vi "Autonomous Independent.vi"() -> ()   [LabVIEW 2011]
doc: "This VI is called when autonomous begins, and will automatically be terminated when autonomous ends. You can carry out timed or sensor driven robot movement independently without needing to return to the caller."
uses:
  <vilib>/Rock Robotics/WPI/Joystick/WPI_JoystickButtonState.ctl
  Robot Global Data.vi
  <vilib>/addons/control/pid/pid.llb/PID (DBL).vi
  <vilib>/Rock Robotics/WPI/RobotDrive/WPI_RobotDriveArcadeDrive_Standard(NoSaturation).vi
  <vilib>/addons/control/pid/NI_PID_pid.lvlib
panel:
  in  "Initial_Delay_Right":u32(slide)=21 scale=0.0..100.0
  in  "Initial_Delay_Left":u32(slide)=1 scale=0.0..100.0
  in  "Initial_Delay_Center":u32(slide)=1 scale=0.0..100.0
  in  "Ball_Sucker_Right":dbl(slide)=0.6 scale=-1.0..1.0
  in  "Ball_Sucker_Left":dbl(slide)=0.6 scale=-1.0..1.0
  in  "Feed_Speed_Right":dbl(slide)=0.9 scale=-1.0..1.0
  in  "Feed_Speed_Left":dbl(slide)=0.9 scale=-1.0..1.0
  in  "Shooter_Speed_ Right":dbl(slide)=0.65 scale=-1.0..1.0
  in  "Shooter_Speed_Left":dbl(slide)=0.365 scale=-1.0..1.0
  in  "Shooting_Time_Left_Position":u32(slide)=25 scale=0.0..100.0
  in  "Forward_Time1_Left_Position":i32(slide)=45 scale=0.0..100.0
  in  "Backward_Time_Left_Position":i32(slide)=70 scale=0.0..100.0
  in  "Turn_Time_Left_Position":i32(slide)=25 scale=0.0..100.0
  in  "Forward_Time2_Left_Position":i32(slide)=15 scale=0.0..100.0
  in  "Shooting_Time_Right_Position":u32(slide)=35 scale=0.0..100.0
  in  "Forward_Time1_Right_Position":i32(slide)=20 scale=0.0..100.0
  in  "Backward_Time_Right_Position":i32(slide)=81 scale=0.0..100.0
  in  "Turn_Time_Right_Position":i32(slide)=25 scale=0.0..100.0
  in  "Forward_Time2_Right_Position":i32(slide)=15 scale=0.0..100.0
  in  "Forward_Time2_Center_Position":i32(slide)=1 scale=0.0..100.0
  in  "Turn_Time_Center_Position":i32(slide)=1 scale=0.0..100.0
  in  "Backward_Time_Center_Position":i32(slide)=51 scale=0.0..100.0
  in  "Forward_Time1_Center_Position":i32(slide)=51 scale=0.0..100.0
  in  "Shooting_Time_Center_Position":u32(slide)=31 scale=0.0..100.0
  in  "Shooter_Speed_Center":dbl(slide)=0.4 scale=-1.0..1.0
  in  "ARM_FWD_LIMIT":dbl(slide)=0.53 scale=1.0..-1.0
  in  "ARM_REV_LIMIT":dbl(slide)=-0.14110429447852763 scale=1.0..-1.0
  in  "ARM_HOME":dbl(slide)=0.53 scale=1.0..-1.0
  in  "Feeder_Arm_Speed":dbl
  out "JS1_BTNS":T1
  out "JS1_AXES":T2
  in  "Kinect_Arm_Conrol":dbl
  out "Kinect_Drive_Reduce":dbl=0.5
  out "KINECT_BTNS":T1
  out "LEFT_ARM_AXES":T2
  out "RIGHT_ARM_AXES":T2
  in  "Ball_Sucker_Center":dbl(slide)=0.6 scale=-1.0..1.0
  in  "Feed_Speed_Center":dbl(slide)=0.9 scale=-1.0..1.0
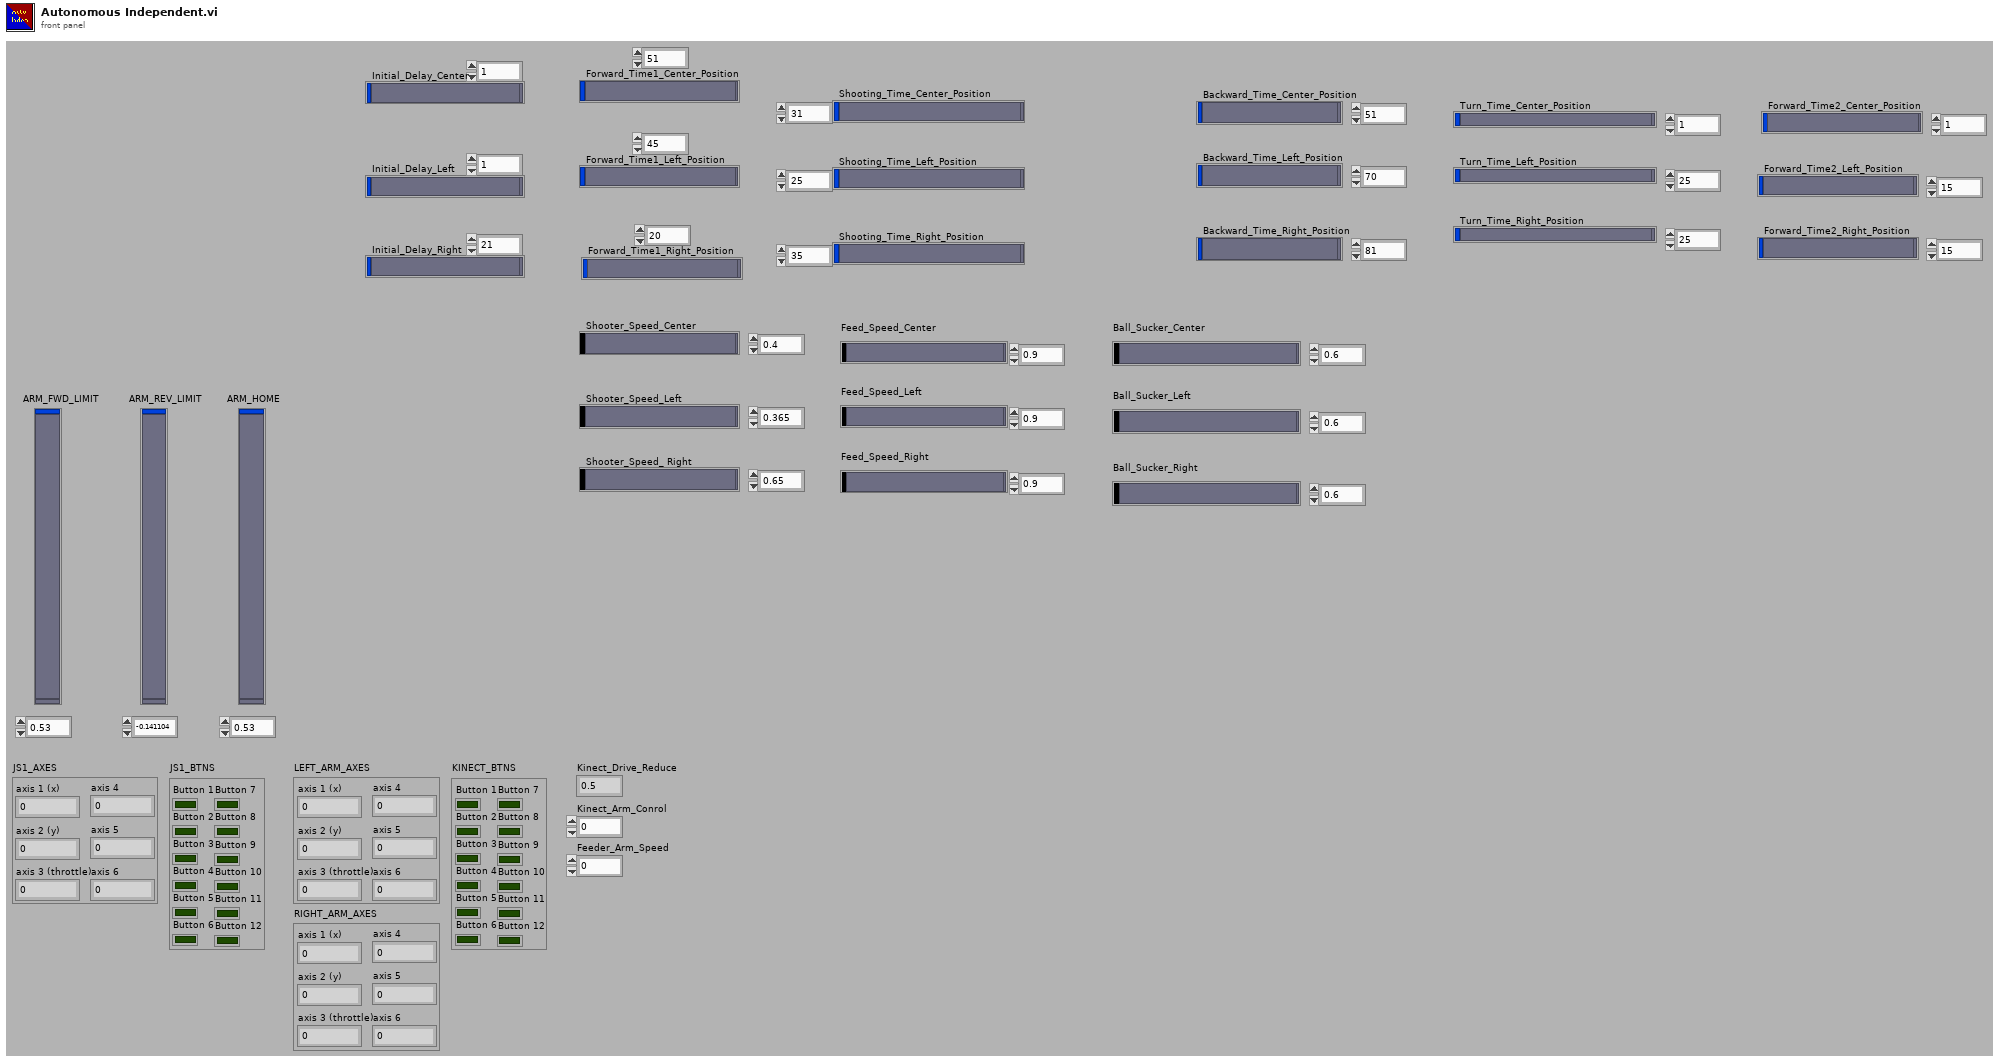
[diagram p1: front panel]
types:
  T1 = typedef "WPI_JoystickButtonState.ctl" = cluster{"Button 1":bool, "Button 2":bool, "Button 3":bool, "Button 4":bool, "Button 5":bool, "Button 6":bool, "Button 7":bool, "Button 8":bool, "Button 9":bool, "Button 10":bool, "Button 11":bool, "Button 12":bool}
  T2 = cluster{"axis 1 (x)":dbl, "axis 2 (y)":dbl, "axis 3 (throttle)":dbl, "axis 4":dbl, "axis 5":dbl, "axis 6":dbl}
  T3 = cluster{"proportional gain (Kc)":dbl, "integral time (Ti, min)":dbl, "derivative time (Td, min)":dbl}
  T4 = typedef "WPI_MotorControlDeviceRef.ctl" = cluster{"DeviceStatus":errorcluster, "Type":enum16{"PWM", "CAN"}, "PWM":cluster{"Digital Module":T5, "PWM Channel":T6, "DeadBand":T7}, "CAN":cluster{"Device Number":u8, "Control Mode":T8, "Semaphore":T9, "Max Vout":dbl}, "Invert":bool, "TransformRef":T10, "InvTransformRef":T10}
  T5 = typedef "FPGA_TypedefDigitalModule.ctl" = enum16{"Digital Module 1", "Digital Module 2"}
  T6 = typedef "FPGA_DIOPWMChannel.ctl" = enum8{"PWM 1", "PWM 2", "PWM 3", "PWM 4", "PWM 5", "PWM 6", "PWM 7", "PWM 8", "PWM 9", "PWM 10", "Invalid"}
  T7 = typedef "WPI_PWMDeadband.ctl" = cluster{"Name":string, "maxPositivePwm":i32, "minPositivePwm":i32, "centerPwm":i32, "maxNegativePwm":i32, "minNegativePwm":i32, "angularRange":u16}
  T8 = typedef "WPI_CANJaguar_ControlMode.ctl" = enum8{"Percent VBus", "Current", "Speed", "Position", "Voltage"}
  T9 = typedef "Semaphore RefNum" = refnum<k1>
  T10 = typedef "WPI_PWMTransform_ConPane.ctl" = refnum<vi>
  T11 = typedef "WPI_RobotDriveDevRef.ctl" = cluster{"DevStatus":errorcluster, "Motors[]":T4[], "Square Inputs":bool, "Max Output":dbl, "Isochronous":bool}
  T12 = typedef "WPI_JoystickDevRef.ctl" = cluster{"Device":T13}
  T13 = typedef "WPI_JoystickDeviceEnum.ctl" = enum16{"USB 1", "USB 2", "USB 3", "USB 4", "Kinect 1", "Kinect 2"}
  T14 = typedef "WPI_AnalogChannelDevRef.ctl" = cluster{"DevStatus":errorcluster, "Analog Module":T15, "Analog Channel":T16}
  T15 = typedef "FPGA_TypedefAnalogModule.ctl" = enum16{"Analog Module 1", "Analog Module 2"}
  T16 = typedef "FPGA_AIChannel.ctl" = enum8{"AI 1", "AI 2", "AI 3", "AI 4", "AI 5", "AI 6", "AI 7", "AI 8", "Invalid"}
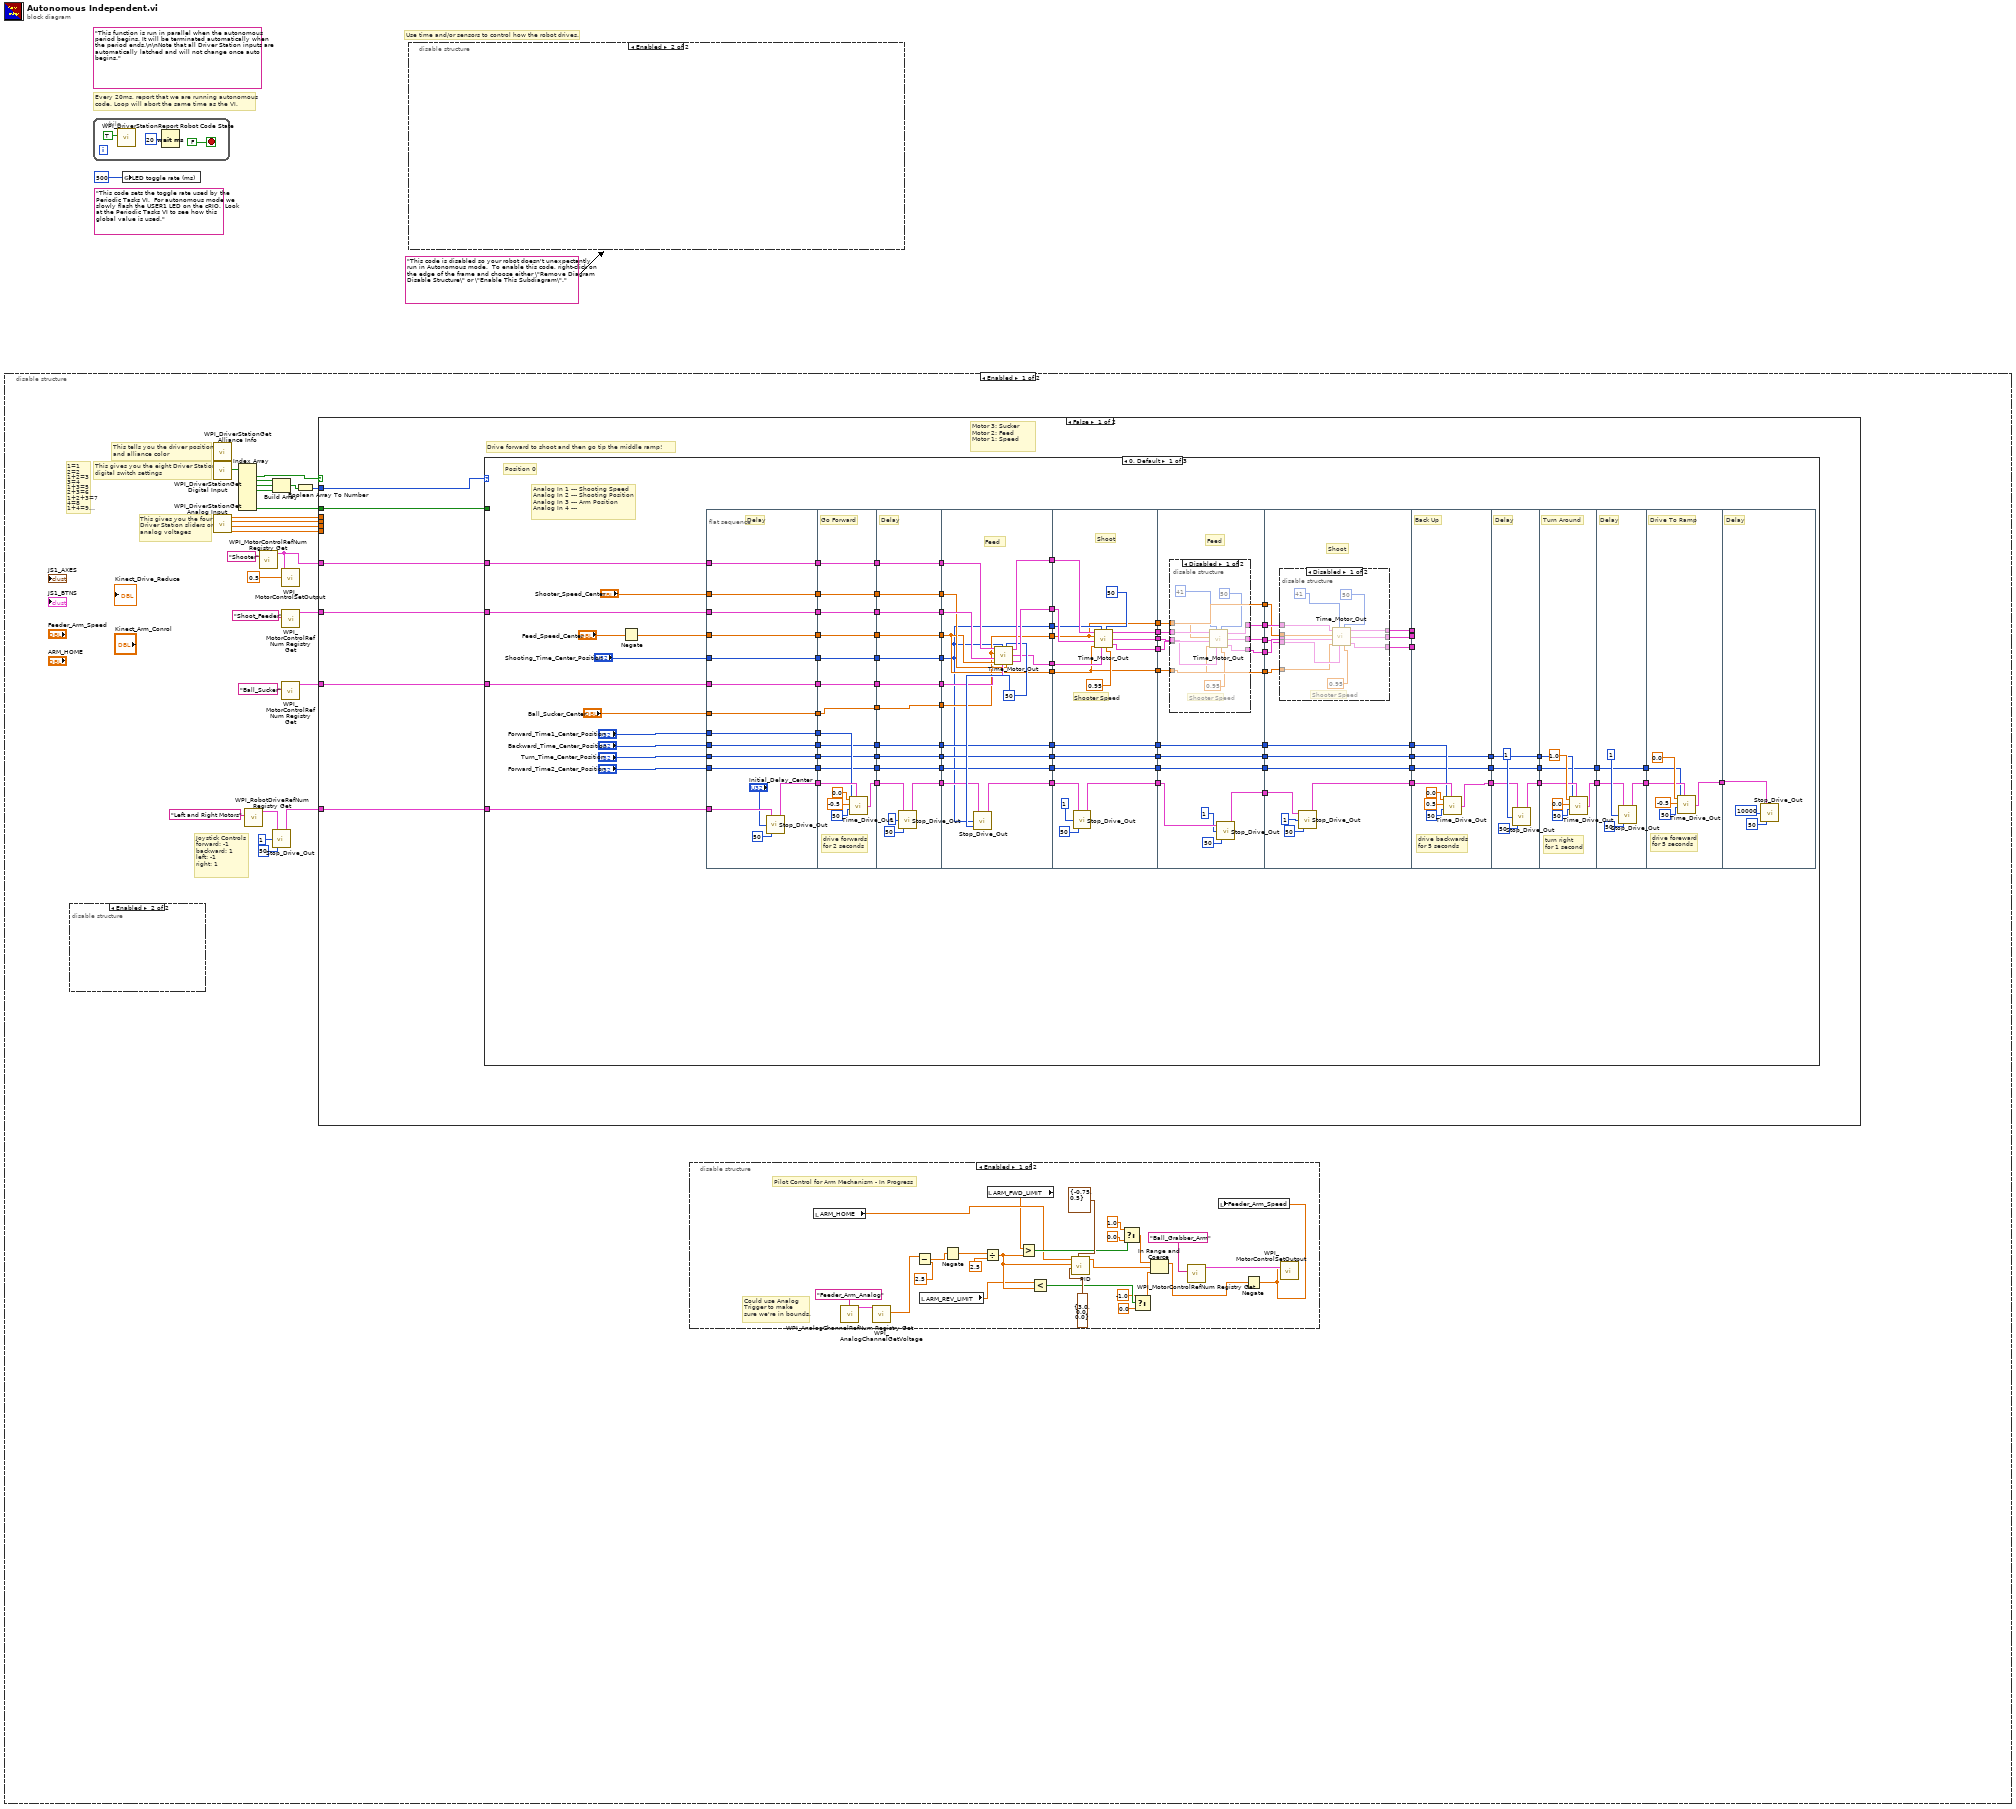
[diagram p0: block diagram]
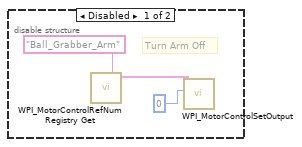
[diagram p3: hidden frame]
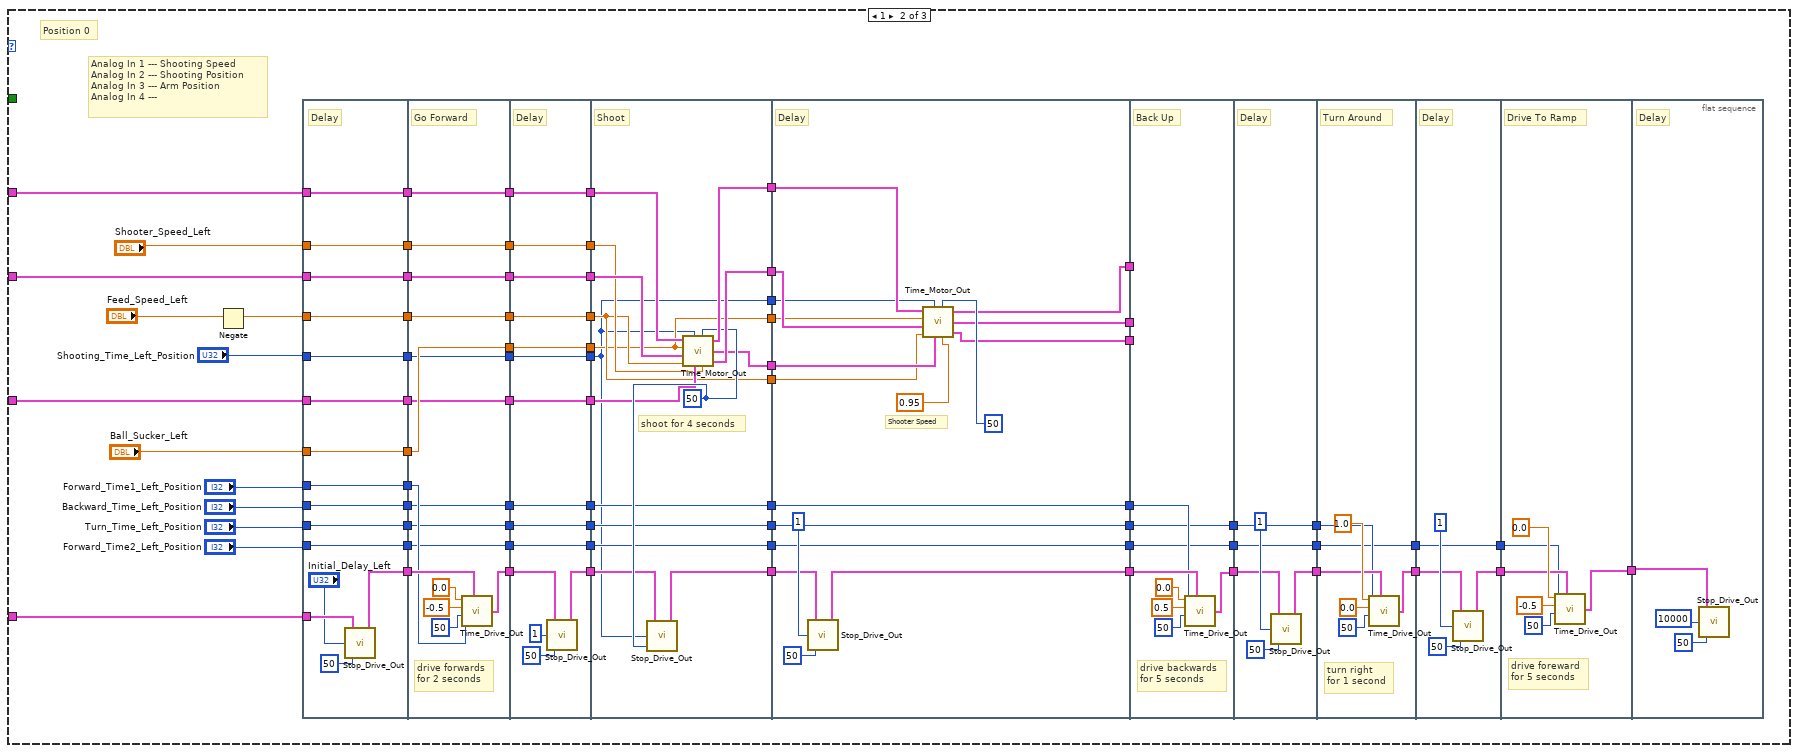
[diagram p6: hidden frame]
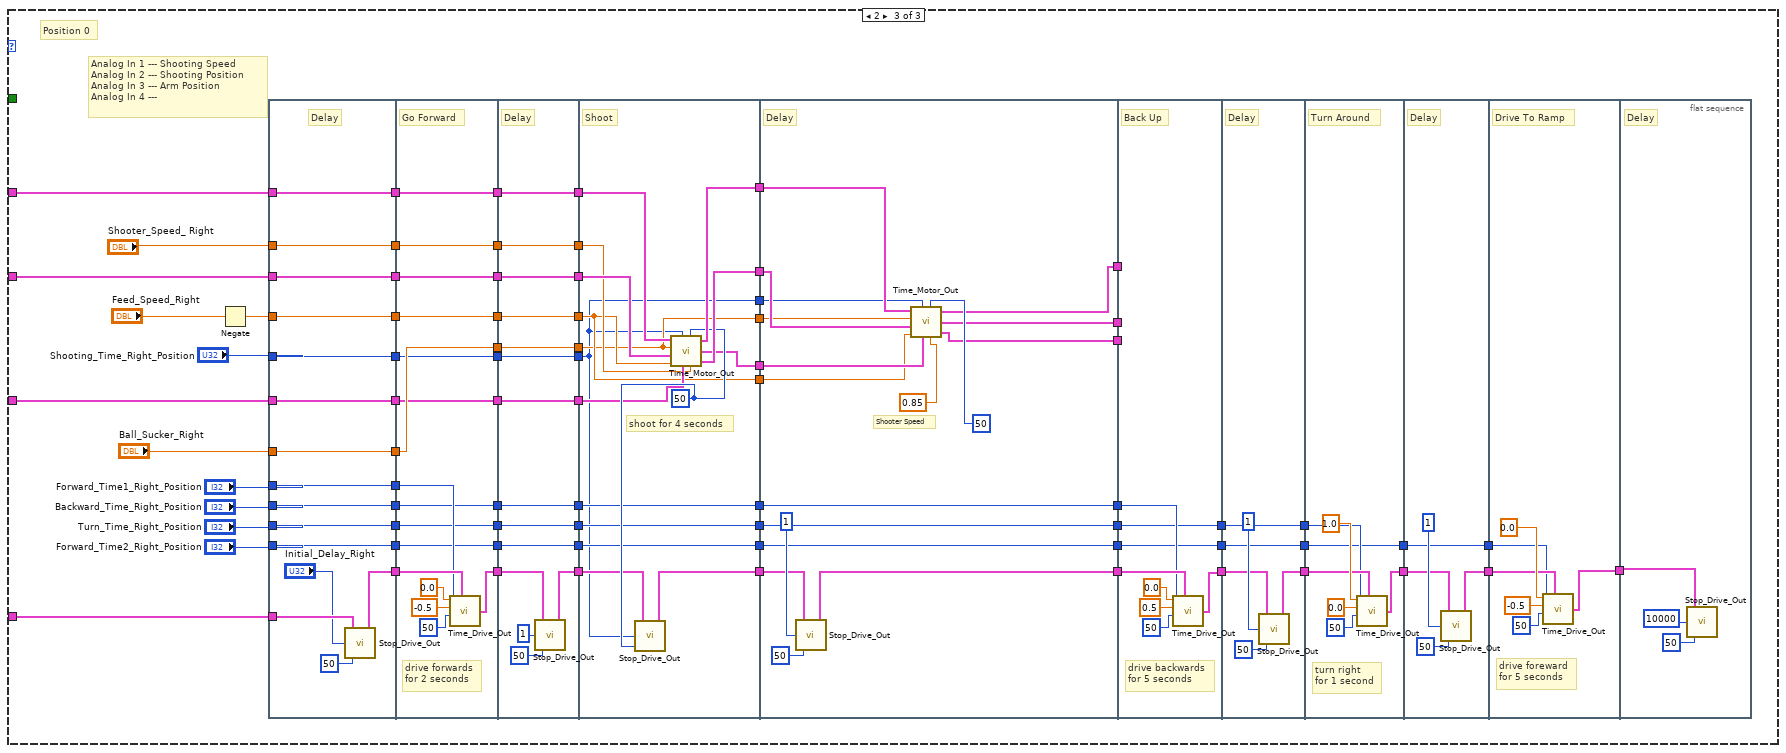
[diagram p7: hidden frame]
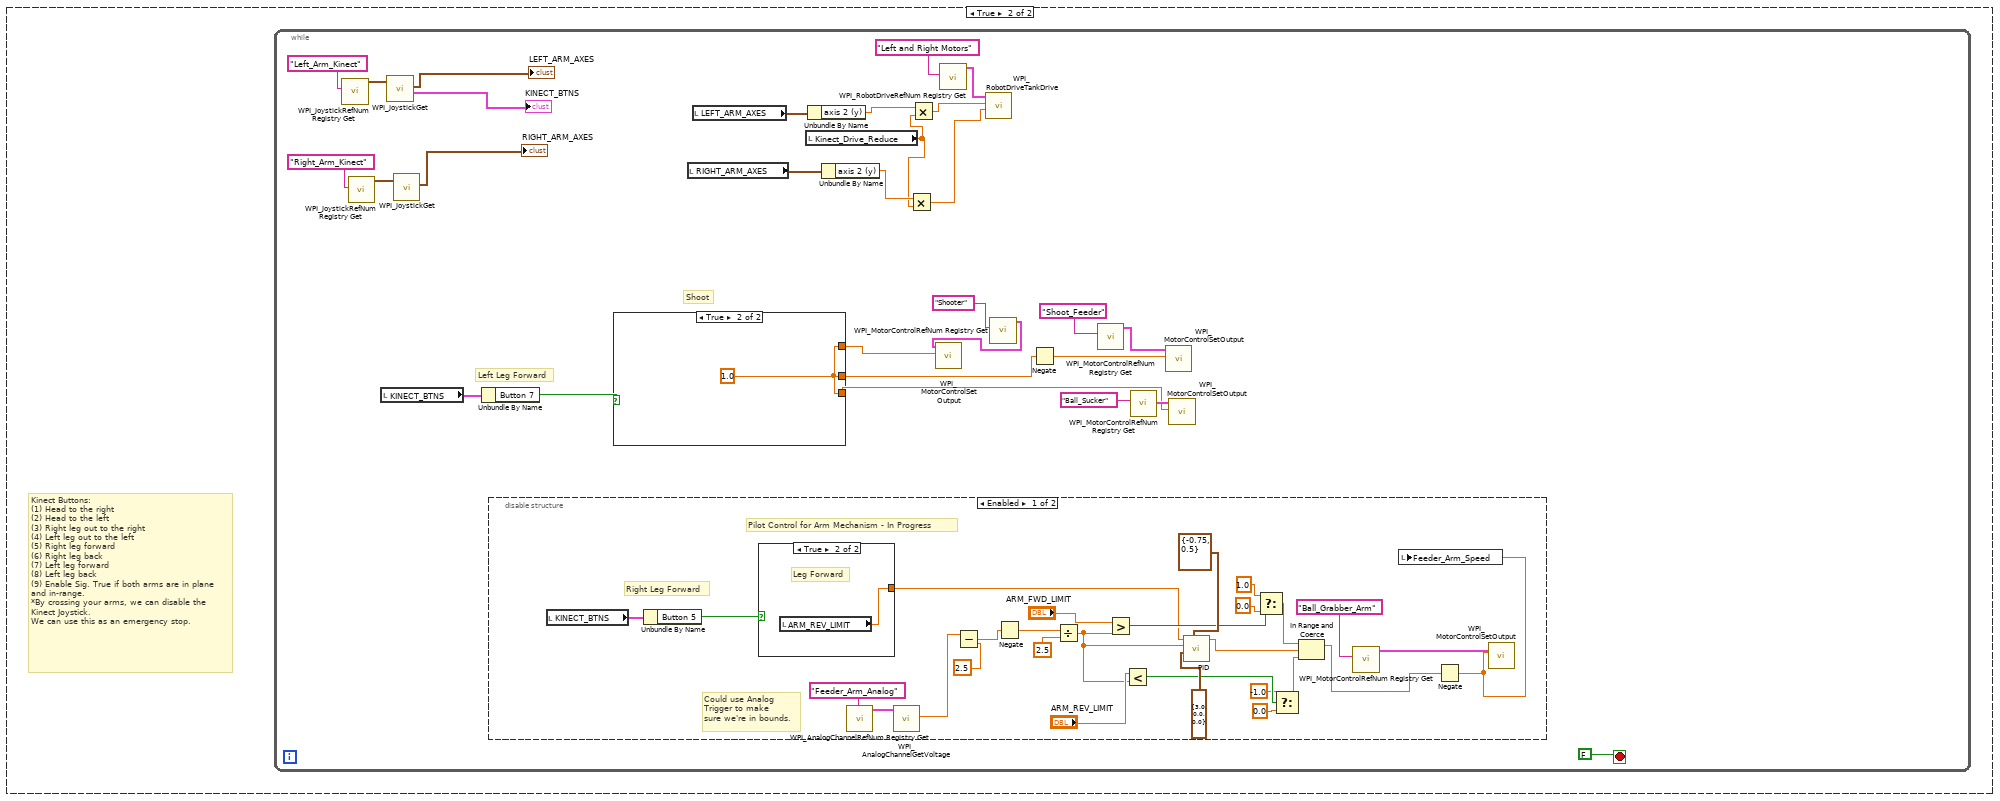
[diagram p8: hidden frame]
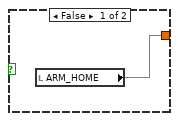
[diagram p9: hidden frame]
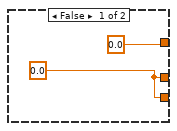
[diagram p11: hidden frame]
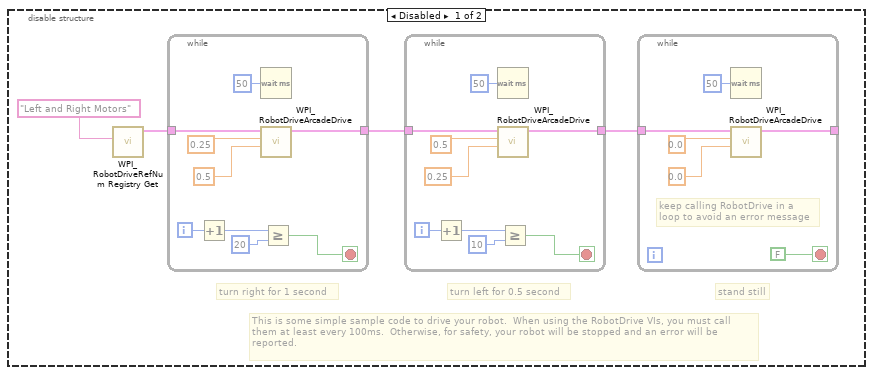
[diagram p13: hidden frame]
diagram:
  (unwired) "This code sets the toggle rate used by the Periodic Tasks VI.  For autonomous mode we slowly flash the USER1 LED on the cRIO.  Look at the Periodic Tasks VI to see how this global value is used."
  (unwired) "This code is disabled so your robot doesn't unexpectantly run in Autonomous mode.  To enable this code, right-click on the edge of the frame and choose either \"Remove Diagram Disable Structure\" or \"Enable This Subdiagram\"."
  (unwired) "This function is run in parallel when the autonomous period begins. It will be terminated automatically when the period ends.\n\nNote that all Driver Station inputs are automatically latched and will not change once auto begins."
  # "Every 20ms, report that we are running autonomous\ncode. Loop will abort the same time as the VI."
  # "Use time and/or sensors to control how the robot drives."
  n1 = disable-structure shown="Enabled" {
    frame Enabled {
      # "Joystick Controls\nforward: -1\nbackward: 1\nleft: -1\nright: 1"
      # "1=1\n2=2\n1+2=3\n3=4\n1+3=5\n2+3=6\n1+2+3=7\n4=8\n1+4=9\n2+4=10\n1+2+4=11\n3+4=12\n1+3+4=13\n2+3+4=14\n1+2+3+4=15"
      # "This tells you the driver position\nand alliance color"
      # "This gives you the eight Driver Station\ndigital switch settings"
      # "This gives you the four\nDriver Station sliders or\nanalog voltages"
      n2 = disable-structure shown="Enabled" {
        frame Disabled {
          # "Turn Arm Off"
          n3 = call <vilib>:"WPI_MotorControlRefNum Registry Get.vi"("refnum name"="Ball_Grabber_Arm") -> ("MotorControlDevRef"=w54:T4)  [unwired: 1 in, 9 out]
          n4 = call <vilib>:"WPI_MotorControlSetOutput.vi"("Output"=0, "MotorControlDevRef"=w54) -> ()  [unwired: 3 in, 7 out]
        }
        frame Enabled {
        }
      }
      n5 = call <vilib>:"WPI_DriverStationGet Alliance Info.vi"() -> ()  [unwired: 12 out]
      n6 = call <vilib>:"WPI_DriverStationGet Digital Input.vi"() -> ("Driver Station Digital Input (1-8)"=w25:bool[])  [unwired: 11 out]
      n7 = call <vilib>:"WPI_DriverStationGet Analog Input.vi"() -> ("Analog 4 (V)"=w22:dbl, "Analog 3 (V)"=w23:dbl, "Analog 2 (V)"=w13:dbl, "Analog 1 (V)"=w14:dbl)  [unwired: 8 out]
      n8 = Index Array(array=w25) -> (element #1=w3:bool, element #2=w2:bool, element #3=w16:bool, element #4=w15:bool, element #8=w21:bool)  [unwired: 8 in, 3 out]
      n9 = call <vilib>:"WPI_RobotDriveRefNum Registry Get.vi"("refnum name"="Left and Right Motors") -> ("RobotDriveDevRef"=w10:T11)  [unwired: 1 in, 9 out]
      n10 = call <vilib>:"WPI_MotorControlRefNum Registry Get.vi"("refnum name"="Shooter") -> ("MotorControlDevRef"=w5:T4)  [unwired: 9 in, 1 out]
      n11 = call "Stop_Drive_Out.vi"("Step_Duration_ms"=50, "Num_Steps"=u32 1 ("milliseconds to wait"), "Drive_In"=w10) -> ("Drive_Out"=w9:T11)
      n12 = Build Array(w2, w16, w15) -> (w24:bool[])
      n13 = call <vilib>:"WPI_MotorControlSetOutput.vi"("Output"=0.5, "MotorControlDevRef"=w5) -> ()  [unwired: 8 in, 2 out]
      n14 = call <vilib>:"WPI_MotorControlRefNum Registry Get.vi"("refnum name"="Ball_Sucker") -> ("MotorControlDevRef"=w6:T4)  [unwired: 9 in, 1 out]
      n15 = call <vilib>:"WPI_MotorControlRefNum Registry Get.vi"("refnum name"="Shoot_Feeder") -> ("MotorControlDevRef"=w18:T4)  [unwired: 9 in, 1 out]
      n16 = Boolean Array To Number(Boolean array=w24) -> (number=w8:u32)
      n17 = case shown="False" w3 {
        tunnel: w14 -> [_ _]
        tunnel: w13 -> [_ _]
        tunnel: w23 -> [_ _]
        tunnel: w22 -> [_ _]
        tunnel: w21 -> [w60 _]
        tunnel: w5 -> [w59 _]
        tunnel: w18 -> [w58 _]
        tunnel: w9 -> [w57 _]
        tunnel: w8 -> [w56 _]
        tunnel: w6 -> [w55 _]
        frame False {
          # "Motor 3: Sucker\nMotor 2: Feed\nMotor 1: Speed"
          # "Drive forward to shoot and then go tip the middle ramp!"
          n18 = case shown="0, Default" w56 {
            tunnel: w60 -> [_ _ _]
            tunnel: w59 -> [w153 w394 w583]
            tunnel: w58 -> [w152 w393 w582]
            tunnel: w57 -> [w151 w392 w581]
            tunnel: w55 -> [w150 w391 w580]
            frame 0, Default {
              # "Analog In 1 --- Shooting Speed\nAnalog In 2 --- Shooting Position\nAnalog In 3 --- Arm Position\nAnalog In 4 ---"
              # "Position 0"
              n19 = Negate(x="Feed_Speed_Center") -> (-x=w88:dbl)
              n20 = flat-sequence {
                tunnel: [w163] -> w149
                tunnel: [w168] -> w148
                tunnel: [w167] -> w147
                tunnel: [w166] -> w146
                tunnel: [w165] -> w145
                tunnel: w153 -> [w166]
                tunnel: w152 -> [w167]
                tunnel: "Shooter_Speed_Center" -> [w165]
                tunnel: w88 -> [w168]
                tunnel: w151 -> [w162]
                tunnel: [w161] -> w144
                tunnel: "Ball_Sucker_Center" -> [w161]
                tunnel: [w160] -> w143
                tunnel: w150 -> [w160]
                tunnel: [w158] -> w117
                tunnel: "Shooting_Time_Center_Position" -> [w158]
                tunnel: "Forward_Time1_Center_Position" -> [w157]
                tunnel: [w157] -> w116
                tunnel: "Backward_Time_Center_Position" -> [w156]
                tunnel: [w156] -> w115
                tunnel: "Turn_Time_Center_Position" -> [w155]
                tunnel: [w155] -> w106
                tunnel: [w154] -> w103
                tunnel: "Forward_Time2_Center_Position" -> [w154]
                tunnel: w149 -> [w181]
                tunnel: [w180] -> w142
                tunnel: [w179] -> w141
                tunnel: w148 -> [w179]
                tunnel: [w178] -> w140
                tunnel: w147 -> [w178]
                tunnel: [w177] -> w139
                tunnel: w146 -> [w177]
                tunnel: [w176] -> w138
                tunnel: w145 -> [w176]
                tunnel: w144 -> [w175]
                tunnel: [w175] -> w137
                tunnel: w143 -> [w174]
                tunnel: [w174] -> w136
                tunnel: [w173] -> w118
                tunnel: w117 -> [w173]
                tunnel: w116 -> [w172]
                tunnel: w115 -> [w171]
                tunnel: [w171] -> w114
                tunnel: [w170] -> w107
                tunnel: w106 -> [w170]
                tunnel: [w169] -> w104
                tunnel: w103 -> [w169]
                tunnel: w142 -> [w192]
                tunnel: [w191] -> w135
                tunnel: [w198] -> w134
                tunnel: w141 -> [w198]
                tunnel: [w197] -> w133
                tunnel: w140 -> [w197]
                tunnel: [w196] -> w132
                tunnel: w139 -> [w196]
                tunnel: [w195] -> w131
                tunnel: w138 -> [w195]
                tunnel: [w190] -> w130
                tunnel: w137 -> [w190]
                tunnel: [w189] -> w129
                tunnel: w136 -> [w189]
                tunnel: [w188] -> w119
                tunnel: w118 -> [w188]
                tunnel: w114 -> [w187]
                tunnel: [w187] -> w113
                tunnel: [w186] -> w108
                tunnel: w107 -> [w186]
                tunnel: [w185] -> w105
                tunnel: w104 -> [w185]
                tunnel: w135 -> [w209]
                tunnel: [w208] -> w128
                tunnel: w134 -> [w201]
                tunnel: w133 -> [w214]
                tunnel: [w213] -> w127
                tunnel: [w212] -> w126
                tunnel: w132 -> [w211]
                tunnel: w131 -> [w205]
                tunnel: [w207] -> w125
                tunnel: w130 -> [w200]
                tunnel: w129 -> [w206]
                tunnel: w119 -> [w199]
                tunnel: w113 -> [w204]
                tunnel: [w204] -> w112
                tunnel: [w203] -> w109
                tunnel: w108 -> [w203]
                tunnel: w105 -> [w202]
                tunnel: [w202] -> w98
                tunnel: [w201] -> w92
                tunnel: [w200] -> w91
                tunnel: [w199] -> w90
                tunnel: w128 -> [w230]
                tunnel: [w229] -> w85
                tunnel: w127 -> [w223]
                tunnel: w126 -> [w224]
                tunnel: w125 -> [w222]
                tunnel: w112 -> [w228]
                tunnel: [w228] -> w84
                tunnel: [w227] -> w83
                tunnel: w109 -> [w227]
                tunnel: [w226] -> w82
                tunnel: w98 -> [w226]
                tunnel: [w221] -> w81
                tunnel: [w220] -> w80
                tunnel: w92 -> [w216]
                tunnel: w91 -> [w215]
                tunnel: w90 -> [w219]
                tunnel: [w217] -> w71
                tunnel: [w216] -> w64
                tunnel: [w215] -> w62
                tunnel: w85 -> [w243]
                tunnel: w84 -> [w247]
                tunnel: [w247] -> w78
                tunnel: w83 -> [w246]
                tunnel: [w246] -> w76
                tunnel: w82 -> [w245]
                tunnel: [w245] -> w74
                tunnel: w81 -> [w235]
                tunnel: w80 -> [w239]
                tunnel: [w241] -> w72
                tunnel: w71 -> [w240]
                tunnel: [w238] -> w70
                tunnel: [w237] -> w69
                tunnel: [w236] -> w68
                tunnel: w64 -> [w234]
                tunnel: [w234] -> w63
                tunnel: w62 -> [w233]
                tunnel: [w233] -> w61
                tunnel: [w268] -> w79
                tunnel: w78 -> [w273]
                tunnel: [w273] -> w77
                tunnel: w76 -> [w272]
                tunnel: [w272] -> w75
                tunnel: w74 -> [w271]
                tunnel: [w271] -> w73
                tunnel: w72 -> [w269]
                tunnel: w70 -> [w266]
                tunnel: w69 -> [w264]
                tunnel: w68 -> [w265]
                tunnel: [w263] -> w67
                tunnel: [w262] -> w66
                tunnel: [w261] -> w65
                tunnel: w63 -> [w260]
                tunnel: w61 -> [w259]
                tunnel: w79 -> [w289]
                tunnel: [w288] -> w124
                tunnel: w77 -> [w287]
                tunnel: [w286] -> w110
                tunnel: w75 -> [w286]
                tunnel: [w285] -> w99
                tunnel: w73 -> [w285]
                tunnel: w67 -> [_]
                tunnel: w66 -> [_]
                tunnel: w65 -> [_]
                tunnel: w124 -> [w296]
                tunnel: [w295] -> w123
                tunnel: [w294] -> w111
                tunnel: w110 -> [w294]
                tunnel: [w293] -> w100
                tunnel: w99 -> [w293]
                tunnel: [w301] -> w122
                tunnel: w123 -> [w302]
                tunnel: w111 -> [w300]
                tunnel: [w299] -> w101
                tunnel: w100 -> [w299]
                tunnel: w122 -> [w308]
                tunnel: [w307] -> w121
                tunnel: [w306] -> w102
                tunnel: w101 -> [w306]
                tunnel: w121 -> [w313]
                tunnel: [w312] -> w120
                tunnel: w102 -> [w311]
                tunnel: w120 -> [w317]
                frame #0 {
                  # "Delay"
                  n21 = call "Stop_Drive_Out.vi"("Step_Duration_ms"=50, "Num_Steps"="Initial_Delay_Center", "Drive_In"=w162) -> ("Drive_Out"=w163:T11)
                }
                frame #1 {
                  # "drive forwards\nfor 2 seconds"
                  # "Go Forward"
                  n22 = call "Time_Drive_Out.vi"("X_Axis"=0.0 ("X axis value"), "Y_Axis"=-0.5 ("X axis value"), "Step_Duration_ms"=u32 50 ("milliseconds to wait"), "Num_Steps"=w172, "Drive_In"=w181) -> ("Drive_Out"=w180:T11)
                }
                frame #2 {
                  # "Delay"
                  n23 = call "Stop_Drive_Out.vi"("Step_Duration_ms"=50, "Num_Steps"=u32 1 ("milliseconds to wait"), "Drive_In"=w192) -> ("Drive_Out"=w191:T11)
                }
                frame #3 {
                  w210 = 50
                  # "Feed"
                  n24 = call "Stop_Drive_Out.vi"("Step_Duration_ms"=w210, "Num_Steps"=w199, "Drive_In"=w209) -> ("Drive_Out"=w208:T11)
                  n25 = call "Time_Motor_Out.vi"("Motor_1_Speed"=w205, "Step_Duration_ms"=w210, "Motor_3"=w206, "Motor_2_Speed"=w201, "Motor_2"=w214, "Num_Steps"=w199, "Motor_3_Speed"=w200, "Motor_1"=w211) -> ("Motor_2_Out"=w213:T4, "Motor_3_Out"=w207:T4, "Motor_1_Out"=w212:T4)
                }
                frame #4 {
                  # "Shooter Speed"
                  # "Shoot"
                  n26 = call "Stop_Drive_Out.vi"("Step_Duration_ms"=50, "Num_Steps"=u32 1 ("milliseconds to wait"), "Drive_In"=w230) -> ("Drive_Out"=w229:T11)
                  n27 = call "Time_Motor_Out.vi"("Motor_1_Speed"=0.95, "Step_Duration_ms"=50, "Motor_3"=w222, "Motor_2_Speed"=w216, "Motor_2"=w223, "Num_Steps"=w219, "Motor_3_Speed"=w215, "Motor_1"=w224) -> ("Motor_2_Out"=w220:T4, "Motor_3_Out"=w221:T4, "Motor_1_Out"=w217:T4)
                }
                frame #5 {
                  # "Feed"
                  n28 = disable-structure shown="Disabled" {
                    disable-tunnel: w240 -> [w256 _]
                    disable-tunnel: w239 -> [w255 _]
                    disable-tunnel: [w254 _] -> w238
                    disable-tunnel: [w253 _] -> w237
                    disable-tunnel: [w252 _] -> w236
                    disable-tunnel: w235 -> [w251 _]
                    disable-tunnel: w234 -> [w249 _]
                    disable-tunnel: w233 -> [w248 _]
                    frame Disabled {
                      # "Shooter Speed"
                      n29 = call "Time_Motor_Out.vi"("Motor_1_Speed"=0.95, "Step_Duration_ms"=50, "Motor_3"=w251, "Motor_2_Speed"=w249, "Motor_2"=w255, "Num_Steps"=41, "Motor_3_Speed"=w248, "Motor_1"=w256) -> ("Motor_2_Out"=w252:T4, "Motor_3_Out"=w253:T4, "Motor_1_Out"=w254:T4)
                    }
                    frame Enabled {
                    }
                  }
                  n30 = call "Stop_Drive_Out.vi"("Step_Duration_ms"=50, "Num_Steps"=u32 1 ("milliseconds to wait"), "Drive_In"=w243) -> ("Drive_Out"=w241:T11)
                }
                frame #6 {
                  # "Shoot"
                  n31 = disable-structure shown="Disabled" {
                    disable-tunnel: w266 -> [w282 _]
                    disable-tunnel: w265 -> [w281 _]
                    disable-tunnel: w264 -> [w280 _]
                    disable-tunnel: [w279 _] -> w263
                    disable-tunnel: [w278 _] -> w262
                    disable-tunnel: [w277 _] -> w261
                    disable-tunnel: w260 -> [w275 _]
                    disable-tunnel: w259 -> [w274 _]
                    frame Disabled {
                      # "Shooter Speed"
                      n32 = call "Time_Motor_Out.vi"("Motor_1_Speed"=0.95, "Step_Duration_ms"=50, "Motor_3"=w280, "Motor_2_Speed"=w275, "Motor_2"=w281, "Num_Steps"=41, "Motor_3_Speed"=w274, "Motor_1"=w282) -> ("Motor_2_Out"=w278:T4, "Motor_3_Out"=w279:T4, "Motor_1_Out"=w277:T4)
                    }
                    frame Enabled {
                    }
                  }
                  n33 = call "Stop_Drive_Out.vi"("Step_Duration_ms"=50, "Num_Steps"=u32 1 ("milliseconds to wait"), "Drive_In"=w269) -> ("Drive_Out"=w268:T11)
                }
                frame #7 {
                  # "Back Up"
                  # "drive backwards\nfor 5 seconds"
                  n34 = call "Time_Drive_Out.vi"("X_Axis"=0.0 ("X axis value"), "Y_Axis"=0.5 ("X axis value"), "Step_Duration_ms"=u32 50 ("milliseconds to wait"), "Num_Steps"=w287, "Drive_In"=w289) -> ("Drive_Out"=w288:T11)
                }
                frame #8 {
                  # "Delay"
                  n35 = call "Stop_Drive_Out.vi"("Step_Duration_ms"=50, "Num_Steps"=u32 1 ("milliseconds to wait"), "Drive_In"=w296) -> ("Drive_Out"=w295:T11)
                }
                frame #9 {
                  # "turn right\nfor 1 second"
                  # "Turn Around"
                  n36 = call "Time_Drive_Out.vi"("X_Axis"=1.0 ("X axis value"), "Y_Axis"=0.0 ("X axis value"), "Step_Duration_ms"=u32 50 ("milliseconds to wait"), "Num_Steps"=w300, "Drive_In"=w302) -> ("Drive_Out"=w301:T11)
                }
                frame #10 {
                  # "Delay"
                  n37 = call "Stop_Drive_Out.vi"("Step_Duration_ms"=50, "Num_Steps"=u32 1 ("milliseconds to wait"), "Drive_In"=w308) -> ("Drive_Out"=w307:T11)
                }
                frame #11 {
                  # "drive foreward\nfor 5 seconds"
                  # "Drive To Ramp"
                  n38 = call "Time_Drive_Out.vi"("X_Axis"=0.0 ("X axis value"), "Y_Axis"=-0.5 ("X axis value"), "Step_Duration_ms"=u32 50 ("milliseconds to wait"), "Num_Steps"=w311, "Drive_In"=w313) -> ("Drive_Out"=w312:T11)
                }
                frame #12 {
                  # "Delay"
                  n39 = call "Stop_Drive_Out.vi"("Step_Duration_ms"=50, "Num_Steps"=u32 10000 ("milliseconds to wait"), "Drive_In"=w317) -> ()  [unwired: 1 out]
                }
              }
            }
            frame 1 {
              # "Analog In 1 --- Shooting Speed\nAnalog In 2 --- Shooting Position\nAnalog In 3 --- Arm Position\nAnalog In 4 ---"
              # "Position 0"
              n40 = Negate(x="Feed_Speed_Left") -> (-x=w320:dbl)
              n41 = flat-sequence {
                tunnel: [w404] -> w390
                tunnel: [w409] -> w389
                tunnel: [w408] -> w388
                tunnel: [w407] -> w387
                tunnel: [w406] -> w386
                tunnel: w394 -> [w407]
                tunnel: w393 -> [w408]
                tunnel: "Shooter_Speed_Left" -> [w406]
                tunnel: w320 -> [w409]
                tunnel: w392 -> [w403]
                tunnel: [w402] -> w385
                tunnel: "Ball_Sucker_Left" -> [w402]
                tunnel: [w401] -> w384
                tunnel: w391 -> [w401]
                tunnel: [w400] -> w357
                tunnel: "Shooting_Time_Left_Position" -> [w400]
                tunnel: "Forward_Time1_Left_Position" -> [w399]
                tunnel: [w399] -> w356
                tunnel: "Backward_Time_Left_Position" -> [w398]
                tunnel: [w398] -> w355
                tunnel: "Turn_Time_Left_Position" -> [w397]
                tunnel: [w397] -> w344
                tunnel: [w396] -> w341
                tunnel: "Forward_Time2_Left_Position" -> [w396]
                tunnel: w390 -> [w422]
                tunnel: [w421] -> w383
                tunnel: [w420] -> w382
                tunnel: w389 -> [w420]
                tunnel: [w419] -> w381
                tunnel: w388 -> [w419]
                tunnel: [w418] -> w380
                tunnel: w387 -> [w418]
                tunnel: [w417] -> w379
                tunnel: w386 -> [w417]
                tunnel: w385 -> [w416]
                tunnel: [w416] -> w378
                tunnel: w384 -> [w415]
                tunnel: [w415] -> w377
                tunnel: [w414] -> w358
                tunnel: w357 -> [w414]
                tunnel: w356 -> [w413]
                tunnel: w355 -> [w412]
                tunnel: [w412] -> w354
                tunnel: [w411] -> w345
                tunnel: w344 -> [w411]
                tunnel: [w410] -> w342
                tunnel: w341 -> [w410]
                tunnel: w383 -> [w433]
                tunnel: [w432] -> w376
                tunnel: [w439] -> w375
                tunnel: w382 -> [w439]
                tunnel: [w438] -> w374
                tunnel: w381 -> [w438]
                tunnel: [w437] -> w373
                tunnel: w380 -> [w437]
                tunnel: [w436] -> w372
                tunnel: w379 -> [w436]
                tunnel: [w431] -> w371
                tunnel: w378 -> [w431]
                tunnel: [w430] -> w370
                tunnel: w377 -> [w430]
                tunnel: [w429] -> w359
                tunnel: w358 -> [w429]
                tunnel: w354 -> [w428]
                tunnel: [w428] -> w353
                tunnel: [w427] -> w346
                tunnel: w345 -> [w427]
                tunnel: [w426] -> w343
                tunnel: w342 -> [w426]
                tunnel: w376 -> [w450]
                tunnel: [w449] -> w369
                tunnel: w375 -> [w442]
                tunnel: w374 -> [w455]
                tunnel: [w454] -> w368
                tunnel: [w453] -> w367
                tunnel: w373 -> [w452]
                tunnel: w372 -> [w446]
                tunnel: [w448] -> w366
                tunnel: w371 -> [w441]
                tunnel: w370 -> [w447]
                tunnel: w359 -> [w440]
                tunnel: w353 -> [w445]
                tunnel: [w445] -> w352
                tunnel: [w444] -> w347
                tunnel: w346 -> [w444]
                tunnel: w343 -> [w443]
                tunnel: [w443] -> w335
                tunnel: [w442] -> w326
                tunnel: [w441] -> w325
                tunnel: [w440] -> w324
                tunnel: w369 -> [w471]
                tunnel: [w470] -> w365
                tunnel: w368 -> [w464]
                tunnel: w367 -> [w465]
                tunnel: w366 -> [w463]
                tunnel: w352 -> [w469]
                tunnel: [w469] -> w351
                tunnel: [w468] -> w348
                tunnel: w347 -> [w468]
                tunnel: [w467] -> w336
                tunnel: w335 -> [w467]
                tunnel: [w462] -> w329
                tunnel: [w461] -> w328
                tunnel: [w460] -> w327
                tunnel: w326 -> [w459]
                tunnel: w325 -> [w458]
                tunnel: w324 -> [w457]
                tunnel: w365 -> [w478]
                tunnel: [w477] -> w364
                tunnel: w351 -> [w476]
                tunnel: [w475] -> w349
                tunnel: w348 -> [w475]
                tunnel: [w474] -> w337
                tunnel: w336 -> [w474]
                tunnel: w329 -> [_]
                tunnel: w328 -> [_]
                tunnel: w327 -> [_]
                tunnel: w364 -> [w485]
                tunnel: [w484] -> w363
                tunnel: [w483] -> w350
                tunnel: w349 -> [w483]
                tunnel: [w482] -> w338
                tunnel: w337 -> [w482]
                tunnel: [w490] -> w362
                tunnel: w363 -> [w491]
                tunnel: w350 -> [w489]
                tunnel: [w488] -> w339
                tunnel: w338 -> [w488]
                tunnel: w362 -> [w497]
                tunnel: [w496] -> w361
                tunnel: [w495] -> w340
                tunnel: w339 -> [w495]
                tunnel: w361 -> [w502]
                tunnel: [w501] -> w360
                tunnel: w340 -> [w500]
                tunnel: w360 -> [w506]
                frame #0 {
                  # "Delay"
                  n42 = call "Stop_Drive_Out.vi"("Step_Duration_ms"=50, "Num_Steps"="Initial_Delay_Left", "Drive_In"=w403) -> ("Drive_Out"=w404:T11)
                }
                frame #1 {
                  # "drive forwards\nfor 2 seconds"
                  # "Go Forward"
                  n43 = call "Time_Drive_Out.vi"("X_Axis"=0.0 ("X axis value"), "Y_Axis"=-0.5 ("X axis value"), "Step_Duration_ms"=u32 50 ("milliseconds to wait"), "Num_Steps"=w413, "Drive_In"=w422) -> ("Drive_Out"=w421:T11)
                }
                frame #2 {
                  # "Delay"
                  n44 = call "Stop_Drive_Out.vi"("Step_Duration_ms"=50, "Num_Steps"=u32 1 ("milliseconds to wait"), "Drive_In"=w433) -> ("Drive_Out"=w432:T11)
                }
                frame #3 {
                  w451 = 50
                  # "Shoot"
                  # "shoot for 4 seconds"
                  n45 = call "Stop_Drive_Out.vi"("Step_Duration_ms"=w451, "Num_Steps"=w440, "Drive_In"=w450) -> ("Drive_Out"=w449:T11)
                  n46 = call "Time_Motor_Out.vi"("Motor_1_Speed"=w446, "Step_Duration_ms"=w451, "Motor_3"=w447, "Motor_2_Speed"=w442, "Motor_2"=w455, "Num_Steps"=w440, "Motor_3_Speed"=w441, "Motor_1"=w452) -> ("Motor_2_Out"=w454:T4, "Motor_3_Out"=w448:T4, "Motor_1_Out"=w453:T4)
                }
                frame #4 {
                  # "Shooter Speed"
                  # "Delay"
                  n47 = call "Stop_Drive_Out.vi"("Step_Duration_ms"=50, "Num_Steps"=u32 1 ("milliseconds to wait"), "Drive_In"=w471) -> ("Drive_Out"=w470:T11)
                  n48 = call "Time_Motor_Out.vi"("Motor_1_Speed"=0.95, "Step_Duration_ms"=50, "Motor_3"=w463, "Motor_2_Speed"=w459, "Motor_2"=w464, "Num_Steps"=w457, "Motor_3_Speed"=w458, "Motor_1"=w465) -> ("Motor_2_Out"=w460:T4, "Motor_3_Out"=w461:T4, "Motor_1_Out"=w462:T4)
                }
                frame #5 {
                  # "Back Up"
                  # "drive backwards\nfor 5 seconds"
                  n49 = call "Time_Drive_Out.vi"("X_Axis"=0.0 ("X axis value"), "Y_Axis"=0.5 ("X axis value"), "Step_Duration_ms"=u32 50 ("milliseconds to wait"), "Num_Steps"=w476, "Drive_In"=w478) -> ("Drive_Out"=w477:T11)
                }
                frame #6 {
                  # "Delay"
                  n50 = call "Stop_Drive_Out.vi"("Step_Duration_ms"=50, "Num_Steps"=u32 1 ("milliseconds to wait"), "Drive_In"=w485) -> ("Drive_Out"=w484:T11)
                }
                frame #7 {
                  # "turn right\nfor 1 second"
                  # "Turn Around"
                  n51 = call "Time_Drive_Out.vi"("X_Axis"=1.0 ("X axis value"), "Y_Axis"=0.0 ("X axis value"), "Step_Duration_ms"=u32 50 ("milliseconds to wait"), "Num_Steps"=w489, "Drive_In"=w491) -> ("Drive_Out"=w490:T11)
                }
                frame #8 {
                  # "Delay"
                  n52 = call "Stop_Drive_Out.vi"("Step_Duration_ms"=50, "Num_Steps"=u32 1 ("milliseconds to wait"), "Drive_In"=w497) -> ("Drive_Out"=w496:T11)
                }
                frame #9 {
                  # "drive foreward\nfor 5 seconds"
                  # "Drive To Ramp"
                  n53 = call "Time_Drive_Out.vi"("X_Axis"=0.0 ("X axis value"), "Y_Axis"=-0.5 ("X axis value"), "Step_Duration_ms"=u32 50 ("milliseconds to wait"), "Num_Steps"=w500, "Drive_In"=w502) -> ("Drive_Out"=w501:T11)
                }
                frame #10 {
                  # "Delay"
                  n54 = call "Stop_Drive_Out.vi"("Step_Duration_ms"=50, "Num_Steps"=u32 10000 ("milliseconds to wait"), "Drive_In"=w506) -> ()  [unwired: 1 out]
                }
              }
            }
            frame 2 {
              # "Analog In 1 --- Shooting Speed\nAnalog In 2 --- Shooting Position\nAnalog In 3 --- Arm Position\nAnalog In 4 ---"
              # "Position 0"
              n55 = Negate(x="Feed_Speed_Right") -> (-x=w510:dbl)
              n56 = flat-sequence {
                tunnel: [w593] -> w579
                tunnel: [w598] -> w578
                tunnel: [w597] -> w577
                tunnel: [w596] -> w576
                tunnel: [w595] -> w575
                tunnel: w583 -> [w596]
                tunnel: w582 -> [w597]
                tunnel: "Shooter_Speed_ Right" -> [w595]
                tunnel: w510 -> [w598]
                tunnel: w581 -> [w592]
                tunnel: [w591] -> w574
                tunnel: "Ball_Sucker_Right" -> [w591]
                tunnel: [w590] -> w573
                tunnel: w580 -> [w590]
                tunnel: [w589] -> w546
                tunnel: "Shooting_Time_Right_Position" -> [w589]
                tunnel: "Forward_Time1_Right_Position" -> [w588]
                tunnel: [w588] -> w545
                tunnel: "Backward_Time_Right_Position" -> [w587]
                tunnel: [w587] -> w544
                tunnel: "Turn_Time_Right_Position" -> [w586]
                tunnel: [w586] -> w533
                tunnel: [w585] -> w530
                tunnel: "Forward_Time2_Right_Position" -> [w585]
                tunnel: w579 -> [w611]
                tunnel: [w610] -> w572
                tunnel: [w609] -> w571
                tunnel: w578 -> [w609]
                tunnel: [w608] -> w570
                tunnel: w577 -> [w608]
                tunnel: [w607] -> w569
                tunnel: w576 -> [w607]
                tunnel: [w606] -> w568
                tunnel: w575 -> [w606]
                tunnel: w574 -> [w605]
                tunnel: [w605] -> w567
                tunnel: w573 -> [w604]
                tunnel: [w604] -> w566
                tunnel: [w603] -> w547
                tunnel: w546 -> [w603]
                tunnel: w545 -> [w602]
                tunnel: w544 -> [w601]
                tunnel: [w601] -> w543
                tunnel: [w600] -> w534
                tunnel: w533 -> [w600]
                tunnel: [w599] -> w531
                tunnel: w530 -> [w599]
                tunnel: w572 -> [w622]
                tunnel: [w621] -> w565
                tunnel: [w628] -> w564
                tunnel: w571 -> [w628]
                tunnel: [w627] -> w563
                tunnel: w570 -> [w627]
                tunnel: [w626] -> w562
                tunnel: w569 -> [w626]
                tunnel: [w625] -> w561
                tunnel: w568 -> [w625]
                tunnel: [w620] -> w560
                tunnel: w567 -> [w620]
                tunnel: [w619] -> w559
                tunnel: w566 -> [w619]
                tunnel: [w618] -> w548
                tunnel: w547 -> [w618]
                tunnel: w543 -> [w617]
                tunnel: [w617] -> w542
                tunnel: [w616] -> w535
                tunnel: w534 -> [w616]
                tunnel: [w615] -> w532
                tunnel: w531 -> [w615]
                tunnel: w565 -> [w639]
                tunnel: [w638] -> w558
                tunnel: w564 -> [w631]
                tunnel: w563 -> [w644]
                tunnel: [w643] -> w557
                tunnel: [w642] -> w556
                tunnel: w562 -> [w641]
                tunnel: w561 -> [w635]
                tunnel: [w637] -> w555
                tunnel: w560 -> [w630]
                tunnel: w559 -> [w636]
                tunnel: w548 -> [w629]
                tunnel: w542 -> [w634]
                tunnel: [w634] -> w541
                tunnel: [w633] -> w536
                tunnel: w535 -> [w633]
                tunnel: w532 -> [w632]
                tunnel: [w632] -> w524
                tunnel: [w631] -> w515
                tunnel: [w630] -> w514
                tunnel: [w629] -> w513
                tunnel: w558 -> [w660]
                tunnel: [w659] -> w554
                tunnel: w557 -> [w653]
                tunnel: w556 -> [w654]
                tunnel: w555 -> [w652]
                tunnel: w541 -> [w658]
                tunnel: [w658] -> w540
                tunnel: [w657] -> w537
                tunnel: w536 -> [w657]
                tunnel: [w656] -> w525
                tunnel: w524 -> [w656]
                tunnel: [w651] -> w518
                tunnel: [w650] -> w517
                tunnel: [w649] -> w516
                tunnel: w515 -> [w648]
                tunnel: w514 -> [w647]
                tunnel: w513 -> [w646]
                tunnel: w554 -> [w667]
                tunnel: [w666] -> w553
                tunnel: w540 -> [w665]
                tunnel: [w664] -> w538
                tunnel: w537 -> [w664]
                tunnel: [w663] -> w526
                tunnel: w525 -> [w663]
                tunnel: w518 -> [_]
                tunnel: w517 -> [_]
                tunnel: w516 -> [_]
                tunnel: w553 -> [w674]
                tunnel: [w673] -> w552
                tunnel: [w672] -> w539
                tunnel: w538 -> [w672]
                tunnel: [w671] -> w527
                tunnel: w526 -> [w671]
                tunnel: [w679] -> w551
                tunnel: w552 -> [w680]
                tunnel: w539 -> [w678]
                tunnel: [w677] -> w528
                tunnel: w527 -> [w677]
                tunnel: w551 -> [w686]
                tunnel: [w685] -> w550
                tunnel: [w684] -> w529
                tunnel: w528 -> [w684]
                tunnel: w550 -> [w691]
                tunnel: [w690] -> w549
                tunnel: w529 -> [w689]
                tunnel: w549 -> [w695]
                frame #0 {
                  # "Delay"
                  n57 = call "Stop_Drive_Out.vi"("Step_Duration_ms"=50, "Num_Steps"="Initial_Delay_Right", "Drive_In"=w592) -> ("Drive_Out"=w593:T11)
                }
                frame #1 {
                  # "drive forwards\nfor 2 seconds"
                  # "Go Forward"
                  n58 = call "Time_Drive_Out.vi"("X_Axis"=0.0 ("X axis value"), "Y_Axis"=-0.5 ("X axis value"), "Step_Duration_ms"=u32 50 ("milliseconds to wait"), "Num_Steps"=w602, "Drive_In"=w611) -> ("Drive_Out"=w610:T11)
                }
                frame #2 {
                  # "Delay"
                  n59 = call "Stop_Drive_Out.vi"("Step_Duration_ms"=50, "Num_Steps"=u32 1 ("milliseconds to wait"), "Drive_In"=w622) -> ("Drive_Out"=w621:T11)
                }
                frame #3 {
                  w640 = 50
                  # "Shoot"
                  # "shoot for 4 seconds"
                  n60 = call "Stop_Drive_Out.vi"("Step_Duration_ms"=w640, "Num_Steps"=w629, "Drive_In"=w639) -> ("Drive_Out"=w638:T11)
                  n61 = call "Time_Motor_Out.vi"("Motor_1_Speed"=w635, "Step_Duration_ms"=w640, "Motor_3"=w636, "Motor_2_Speed"=w631, "Motor_2"=w644, "Num_Steps"=w629, "Motor_3_Speed"=w630, "Motor_1"=w641) -> ("Motor_2_Out"=w643:T4, "Motor_3_Out"=w637:T4, "Motor_1_Out"=w642:T4)
                }
                frame #4 {
                  # "Shooter Speed"
                  # "Delay"
                  n62 = call "Stop_Drive_Out.vi"("Step_Duration_ms"=50, "Num_Steps"=u32 1 ("milliseconds to wait"), "Drive_In"=w660) -> ("Drive_Out"=w659:T11)
                  n63 = call "Time_Motor_Out.vi"("Motor_1_Speed"=0.85, "Step_Duration_ms"=50, "Motor_3"=w652, "Motor_2_Speed"=w648, "Motor_2"=w653, "Num_Steps"=w646, "Motor_3_Speed"=w647, "Motor_1"=w654) -> ("Motor_2_Out"=w649:T4, "Motor_3_Out"=w650:T4, "Motor_1_Out"=w651:T4)
                }
                frame #5 {
                  # "Back Up"
                  # "drive backwards\nfor 5 seconds"
                  n64 = call "Time_Drive_Out.vi"("X_Axis"=0.0 ("X axis value"), "Y_Axis"=0.5 ("X axis value"), "Step_Duration_ms"=u32 50 ("milliseconds to wait"), "Num_Steps"=w665, "Drive_In"=w667) -> ("Drive_Out"=w666:T11)
                }
                frame #6 {
                  # "Delay"
                  n65 = call "Stop_Drive_Out.vi"("Step_Duration_ms"=50, "Num_Steps"=u32 1 ("milliseconds to wait"), "Drive_In"=w674) -> ("Drive_Out"=w673:T11)
                }
                frame #7 {
                  # "turn right\nfor 1 second"
                  # "Turn Around"
                  n66 = call "Time_Drive_Out.vi"("X_Axis"=1.0 ("X axis value"), "Y_Axis"=0.0 ("X axis value"), "Step_Duration_ms"=u32 50 ("milliseconds to wait"), "Num_Steps"=w678, "Drive_In"=w680) -> ("Drive_Out"=w679:T11)
                }
                frame #8 {
                  # "Delay"
                  n67 = call "Stop_Drive_Out.vi"("Step_Duration_ms"=50, "Num_Steps"=u32 1 ("milliseconds to wait"), "Drive_In"=w686) -> ("Drive_Out"=w685:T11)
                }
                frame #9 {
                  # "drive foreward\nfor 5 seconds"
                  # "Drive To Ramp"
                  n68 = call "Time_Drive_Out.vi"("X_Axis"=0.0 ("X axis value"), "Y_Axis"=-0.5 ("X axis value"), "Step_Duration_ms"=u32 50 ("milliseconds to wait"), "Num_Steps"=w689, "Drive_In"=w691) -> ("Drive_Out"=w690:T11)
                }
                frame #10 {
                  # "Delay"
                  n69 = call "Stop_Drive_Out.vi"("Step_Duration_ms"=50, "Num_Steps"=u32 10000 ("milliseconds to wait"), "Drive_In"=w695) -> ()  [unwired: 1 out]
                }
              }
            }
          }
        }
        frame True {
          # "Kinect Buttons:\n(1) Head to the right\n(2) Head to the left\n(3) Right leg out to the right\n(4) Left leg out to the left\n(5) Right leg forward\n(6) Right leg back\n(7) Left leg forward\n(8) Left leg back\n(9) Enable Sig. True if both arms are in plane and in-range.\n*By crossing your arms, we can disable the Kinect Joystick. \nWe can use this as an emergency stop."
          n70 = while {
            stop <- FALSE stop-if-true
            # "Left Leg Forward"
            # "Shoot"
            n71 = call <vilib>:"WPI_JoystickRefNum Registry Get.vi"("refnum name"="Left_Arm_Kinect") -> ("JoystickDevRef"=w723:T12)  [unwired: 1 in, 9 out]
            n72 = call <vilib>:"WPI_JoystickRefNum Registry Get.vi"("refnum name"="Right_Arm_Kinect") -> ("JoystickDevRef"=w721:T12)  [unwired: 1 in, 9 out]
            n73 = local read "KINECT_BTNS"() -> (w711:T1)
            n74 = call <vilib>:"WPI_JoystickGet.vi"("JoystickDevRef"=w723) -> ("Buttons"=→"KINECT_BTNS":T1, "Axes"=→"LEFT_ARM_AXES":T2)  [unwired: 1 in, 4 out]
            n75 = call <vilib>:"WPI_JoystickGet.vi"("JoystickDevRef"=w721) -> ("Axes"=→"RIGHT_ARM_AXES":T2)  [unwired: 1 in, 5 out]
            n76 = Unbundle By Name(w711) -> ("Button 7"=w710:bool)
            n77 = disable-structure shown="Enabled" {
              frame Enabled {
                # "Right Leg Forward"
                # "Could use Analog\nTrigger to make \nsure we're in bounds."
                # "Pilot Control for Arm Mechanism - In Progress"
                n78 = local read "KINECT_BTNS"() -> (w729:T1)
                n79 = Unbundle By Name(w729) -> ("Button 5"=w727:bool)
                n80 = case shown="True" w727 {
                  tunnel: [w755 w756] -> w728
                  frame False {
                    n81 = local read "ARM_HOME"() -> (w755:dbl)
                  }
                  frame True {
                    # "Leg Forward"
                    n82 = local read "ARM_REV_LIMIT"() -> (w756:dbl)
                  }
                }
                n83 = call <vilib>:"WPI_AnalogChannelRefNum Registry Get.vi"("refnum name"="Feeder_Arm_Analog") -> ("AIDeviceRef"=w753:T14)  [unwired: 1 in, 9 out]
                n84 = call <vilib>:"WPI_AnalogChannelGetVoltage.vi"("AIDeviceRef"=w753) -> ("Voltage"=w750:dbl)  [unwired: 1 in, 9 out]
                n85 = Subtract(x=w750, y=2.5) -> (x-y=w733:dbl)
                n86 = Negate(x=w733) -> (-x=w734:dbl)
                n87 = Divide(x=w734, y=2.5) -> (x/y=w731:dbl)
                n88 = Greater?(x="ARM_FWD_LIMIT", y=w731) -> (0:w745:bool)
                n89 = Less?(x="ARM_REV_LIMIT", y=w731) -> (x < y?=w747:bool)
                n90 = call-poly <vilib>:"PID.vi"("output range"=cluster{"output low":dbl, "output high":dbl} {"output low"=-0.75, "output high"=0.5}, "PID gains"=T3 {"proportional gain (Kc)"=3.0, "integral time (Ti, min)"=0.0, "derivative time (Td, min)"=0.0}, "process variable"=w731, "setpoint"=w728) -> ("output"=w738:dbl)  [unwired: 2 in, 5 out]
                n91 = Select(t=1.0, s=w745, f=0.0) -> (s? t:f=w743:dbl)
                n92 = Select(t=-1.0, s=w747, f=0.0) -> (s? t:f=w744:dbl)
                n93 = In Range and Coerce(upper limit=w743, x=w738, lower limit=w744) -> (coerced(x)=w730:dbl)  [unwired: 1 out]
                n94 = call <vilib>:"WPI_MotorControlRefNum Registry Get.vi"("refnum name"="Ball_Grabber_Arm") -> ("MotorControlDevRef"=w754:T4)  [unwired: 1 in, 9 out]
                n95 = Negate(x=w730) -> (-x=w735:dbl)
                n96 = local write "Feeder_Arm_Speed"(w735) -> ()
                n97 = call <vilib>:"WPI_MotorControlSetOutput.vi"("Output"=w735, "MotorControlDevRef"=w754) -> ()  [unwired: 3 in, 7 out]
              }
              frame Disabled {
              }
            }
            n98 = case shown="True" w710 {
              tunnel: [0.0 w759] -> w702
              tunnel: [w758 w759] -> w701
              tunnel: [w758 w759] -> w700
              frame False {
                w758 = 0.0
              }
              frame True {
                w759 = 1.0
              }
            }
            n99 = local read "RIGHT_ARM_AXES"() -> (w714:T2)
            n100 = local read "LEFT_ARM_AXES"() -> (w717:T2)
            n101 = local read "Kinect_Drive_Reduce"() -> (w712:dbl)
            n102 = Unbundle By Name(w717) -> ("axis 2 (y)"=w716:dbl)
            n103 = Unbundle By Name(w714) -> ("axis 2 (y)"=w713:dbl)
            n104 = Multiply(x=w713, y=w712) -> (x*y=w698:dbl)
            n105 = Multiply(x=w716, y=w712) -> (x*y=w715:dbl)
            n106 = call <vilib>:"WPI_RobotDriveRefNum Registry Get.vi"("refnum name"="Left and Right Motors") -> ("RobotDriveDevRef"=w718:T11)  [unwired: 1 in, 9 out]
            n107 = call <vilib>:"WPI_RobotDriveTankDrive.vi"("Right axis value"=w698, "Left axis value"=w715, "RobotDriveDevRef"=w718) -> ()  [unwired: 7 in, 2 out]
            n108 = call <vilib>:"WPI_MotorControlRefNum Registry Get.vi"("refnum name"="Shooter") -> ("MotorControlDevRef"=w708:T4)  [unwired: 9 in, 1 out]
            n109 = call <vilib>:"WPI_MotorControlSetOutput.vi"("Output"=w702, "MotorControlDevRef"=w708) -> ()  [unwired: 8 in, 2 out]
            n110 = Negate(x=w701) -> (-x=w705:dbl)
            n111 = call <vilib>:"WPI_MotorControlRefNum Registry Get.vi"("refnum name"="Shoot_Feeder") -> ("MotorControlDevRef"=w706:T4)  [unwired: 9 in, 1 out]
            n112 = call <vilib>:"WPI_MotorControlRefNum Registry Get.vi"("refnum name"="Ball_Sucker") -> ("MotorControlDevRef"=w703:T4)  [unwired: 9 in, 1 out]
            n113 = call <vilib>:"WPI_MotorControlSetOutput.vi"("Output"=w705, "MotorControlDevRef"=w706) -> ()  [unwired: 8 in, 2 out]
            n114 = call <vilib>:"WPI_MotorControlSetOutput.vi"("Output"=w700, "MotorControlDevRef"=w703) -> ()  [unwired: 8 in, 2 out]
          }
        }
      }
      n115 = disable-structure shown="Enabled" {
        frame Enabled {
          # "Could use Analog\nTrigger to make \nsure we're in bounds."
          # "Pilot Control for Arm Mechanism - In Progress"
          n116 = local read "ARM_HOME"() -> (w28:dbl)
          n117 = call <vilib>:"WPI_AnalogChannelRefNum Registry Get.vi"("refnum name"="Feeder_Arm_Analog") -> ("AIDeviceRef"=w50:T14)  [unwired: 1 in, 9 out]
          n118 = call <vilib>:"WPI_AnalogChannelGetVoltage.vi"("AIDeviceRef"=w50) -> ("Voltage"=w47:dbl)  [unwired: 1 in, 9 out]
          n119 = Subtract(x=w47, y=2.5) -> (x-y=w31:dbl)
          n120 = local read "ARM_REV_LIMIT"() -> (w27:dbl)
          n121 = Negate(x=w31) -> (-x=w32:dbl)
          n122 = Divide(x=w32, y=2.5) -> (x/y=w30:dbl)
          n123 = local read "ARM_FWD_LIMIT"() -> (w26:dbl)
          n124 = Greater?(x=w26, y=w30) -> (0:w43:bool)
          n125 = Less?(x=w27, y=w30) -> (x < y?=w44:bool)
          n126 = call-poly <vilib>:"PID.vi"("output range"=cluster{"output low":dbl, "output high":dbl} {"output low"=-0.75, "output high"=0.5}, "PID gains"=T3 {"proportional gain (Kc)"=3.0, "integral time (Ti, min)"=0.0, "derivative time (Td, min)"=0.0}, "process variable"=w30, "setpoint"=w28) -> ("output"=w36:dbl)  [unwired: 2 in, 5 out]
          n127 = Select(t=1.0, s=w43, f=0.0) -> (s? t:f=w41:dbl)
          n128 = Select(t=-1.0, s=w44, f=0.0) -> (s? t:f=w42:dbl)
          n129 = In Range and Coerce(upper limit=w41, x=w36, lower limit=w42) -> (coerced(x)=w29:dbl)  [unwired: 1 out]
          n130 = call <vilib>:"WPI_MotorControlRefNum Registry Get.vi"("refnum name"="Ball_Grabber_Arm") -> ("MotorControlDevRef"=w51:T4)  [unwired: 1 in, 9 out]
          n131 = Negate(x=w29) -> (-x=w33:dbl)
          n132 = local write "Feeder_Arm_Speed"(w33) -> ()
          n133 = call <vilib>:"WPI_MotorControlSetOutput.vi"("Output"=w33, "MotorControlDevRef"=w51) -> ()  [unwired: 3 in, 7 out]
        }
        frame Disabled {
        }
      }
    }
    frame Disabled {
    }
  }
  n134 = while {
    stop <- FALSE stop-if-true
    n135 = call <vilib>:"WPI_DriverStationReport Robot Code State.vi"("Autonomous"=TRUE) -> ()  [unwired: 10 in, 1 out]
    n136 = Wait (ms)(milliseconds to wait=u32 20) -> ()  [unwired: 1 out]
  }
  n137 = global write "Robot Global Data.vi" "LED toggle rate (ms)"(u32 500 ("LED ms toggle rate")) -> ()
  n138 = disable-structure shown="Enabled" {
    frame Disabled {
      # "This is some simple sample code to drive your robot.  When using the RobotDrive VIs, you must call them at least every 100ms.  Otherwise, for safety, your robot will be stopped and an error will be reported."
      # "stand still"
      # "turn left for 0.5 second"
      # "turn right for 1 second"
      n139 = call <vilib>:"WPI_RobotDriveRefNum Registry Get.vi"("refnum name"="Left and Right Motors") -> ("RobotDriveDevRef"=w765:T11)  [unwired: 1 in, 9 out]
      n140 = while {
        tunnel: w765 -> [w790]
        tunnel: [w783] -> w764
        i -> [w786]
        stop <- w784 stop-if-true
        n141 = Increment(x=w786) -> (x+1=w782:i32)
        n142 = Wait (ms)(milliseconds to wait=u32 50) -> ()  [unwired: 1 out]
        n143 = call-poly <vilib>:"WPI_RobotDriveArcadeDrive.vi"("Y axis value"=0.5 ("X axis value"), "X axis value"=0.25, "RobotDriveDevRef"=w790) -> ("RobotDriveDevRef"=w783:T11)  [unwired: 1 in, 7 out]
        n144 = Greater Or Equal?(x=w782, y=20) -> (x >= y?=w784:bool)
      }
      n145 = while {
        tunnel: w764 -> [w781]
        tunnel: [w774] -> w763
        i -> [w777]
        stop <- w775 stop-if-true
        n146 = Increment(x=w777) -> (x+1=w773:i32)
        n147 = Wait (ms)(milliseconds to wait=u32 50) -> ()  [unwired: 1 out]
        n148 = call-poly <vilib>:"WPI_RobotDriveArcadeDrive.vi"("Y axis value"=0.25 ("X axis value"), "X axis value"=0.5, "RobotDriveDevRef"=w781) -> ("RobotDriveDevRef"=w774:T11)  [unwired: 1 in, 7 out]
        n149 = Greater Or Equal?(x=w773, y=10) -> (x >= y?=w775:bool)
      }
      n150 = while {
        tunnel: w763 -> [w772]
        tunnel: [w768] -> _
        stop <- FALSE stop-if-true
        # "keep calling RobotDrive in a loop to avoid an error message"
        n151 = Wait (ms)(milliseconds to wait=u32 50) -> ()  [unwired: 1 out]
        n152 = call-poly <vilib>:"WPI_RobotDriveArcadeDrive.vi"("Y axis value"=0.0 ("X axis value"), "X axis value"=0.0, "RobotDriveDevRef"=w772) -> ("RobotDriveDevRef"=w768:T11)  [unwired: 1 in, 7 out]
      }
    }
    frame Enabled {
    }
  }
